vi "simulator.vi"() -> ()   [LabVIEW 2020]
doc: "This example demonstrates how to continuously acquire buffered voltage measurements using a DAQmx device.\n\nFor instructions on how to connect your signals to the DAQ device, refer to your device documentation."
uses:
  <vilib>/Utility/error.llb/DialogType.ctl
  <vilib>/measure/NI_MAPro.lvlib
  <vilib>/express/express arith-compare/Formula/XNode/ExpressFormulaBlockNode.xnode
  <vilib>/DAQmx/configure/task.llb/DAQmx Configure Logging (TDMS).vi
  <vilib>/measure/maspectr.llb/FFT Power Spectrum and PSD for N Chan.vi
  <vilib>/DAQmx/read.llb/DAQmx Read (Analog 1D Wfm NChan NSamp).vi
  <vilib>/express/express shared/transition.llb/Dynamic To Waveform Array.vi
  <vilib>/express/express arith-compare/Formula/Block/exnFormulaBlock how many pts in the wave.vi
  <vilib>/express/express shared/ex_Modify Signal Name.vi
  <vilib>/express/express shared/transition.llb/Waveform Array To Dynamic.vi
panel:
  in  "라디오 버튼":T1(radio)
  out "Sensor A Raw 6":dynamicdata(graph)
  in  "Sensor C Channel 2":tag="Dev2/ai0"
  in  "Sensor D Channel 2":tag="Dev2/ai1"
  in  "Terminal config 2":i32(ring)=10083 items=["default"=-1, "RSE"=10083, "NRSE"=10078, "Differential"=10106, "Pseudodifferential"=12529]
  out "A,B Filtering Signal 2":dynamicdata(graph)
  out "불리언 5":bool
  out "불리언 4":bool
  out "불리언 3":bool
  out "불리언 2":bool
  out "A,B Filtering Signal":dynamicdata(graph)
  out "Sensor A Raw 5":dynamicdata(graph)
  out "B Raw Signal":waveform(dbl)(graph)
  out "A Raw Signal":waveform(dbl)(graph)
  in  "TDMS File Path":path
  in  "Logging Mode":i32(ring)=10231 items=["Off"=10231, "Log and Read"=15842]
  in  "Sensor B Channel":tag="Dev2/ai1"
  in  "Sensor A Channel":tag="Dev2/ai0"
  in  "Terminal config":i32(ring)=10083 items=["default"=-1, "RSE"=10083, "NRSE"=10078, "Differential"=10106, "Pseudodifferential"=12529]
  in  "rate":dbl=5000.0
  out "FFT Power Spectrum":cluster{"f0":dbl, "df":dbl, "magnitude":dbl[]}[](graph)
  in  "Stop":bool
  in  "Number of Samples":i32=100
  # "A신호"
  # "B신호"
  # "Channel Settings"
  # "A신호"
  # "B신호"
  # "Logging Settings"
  # "A-B Signal Display"
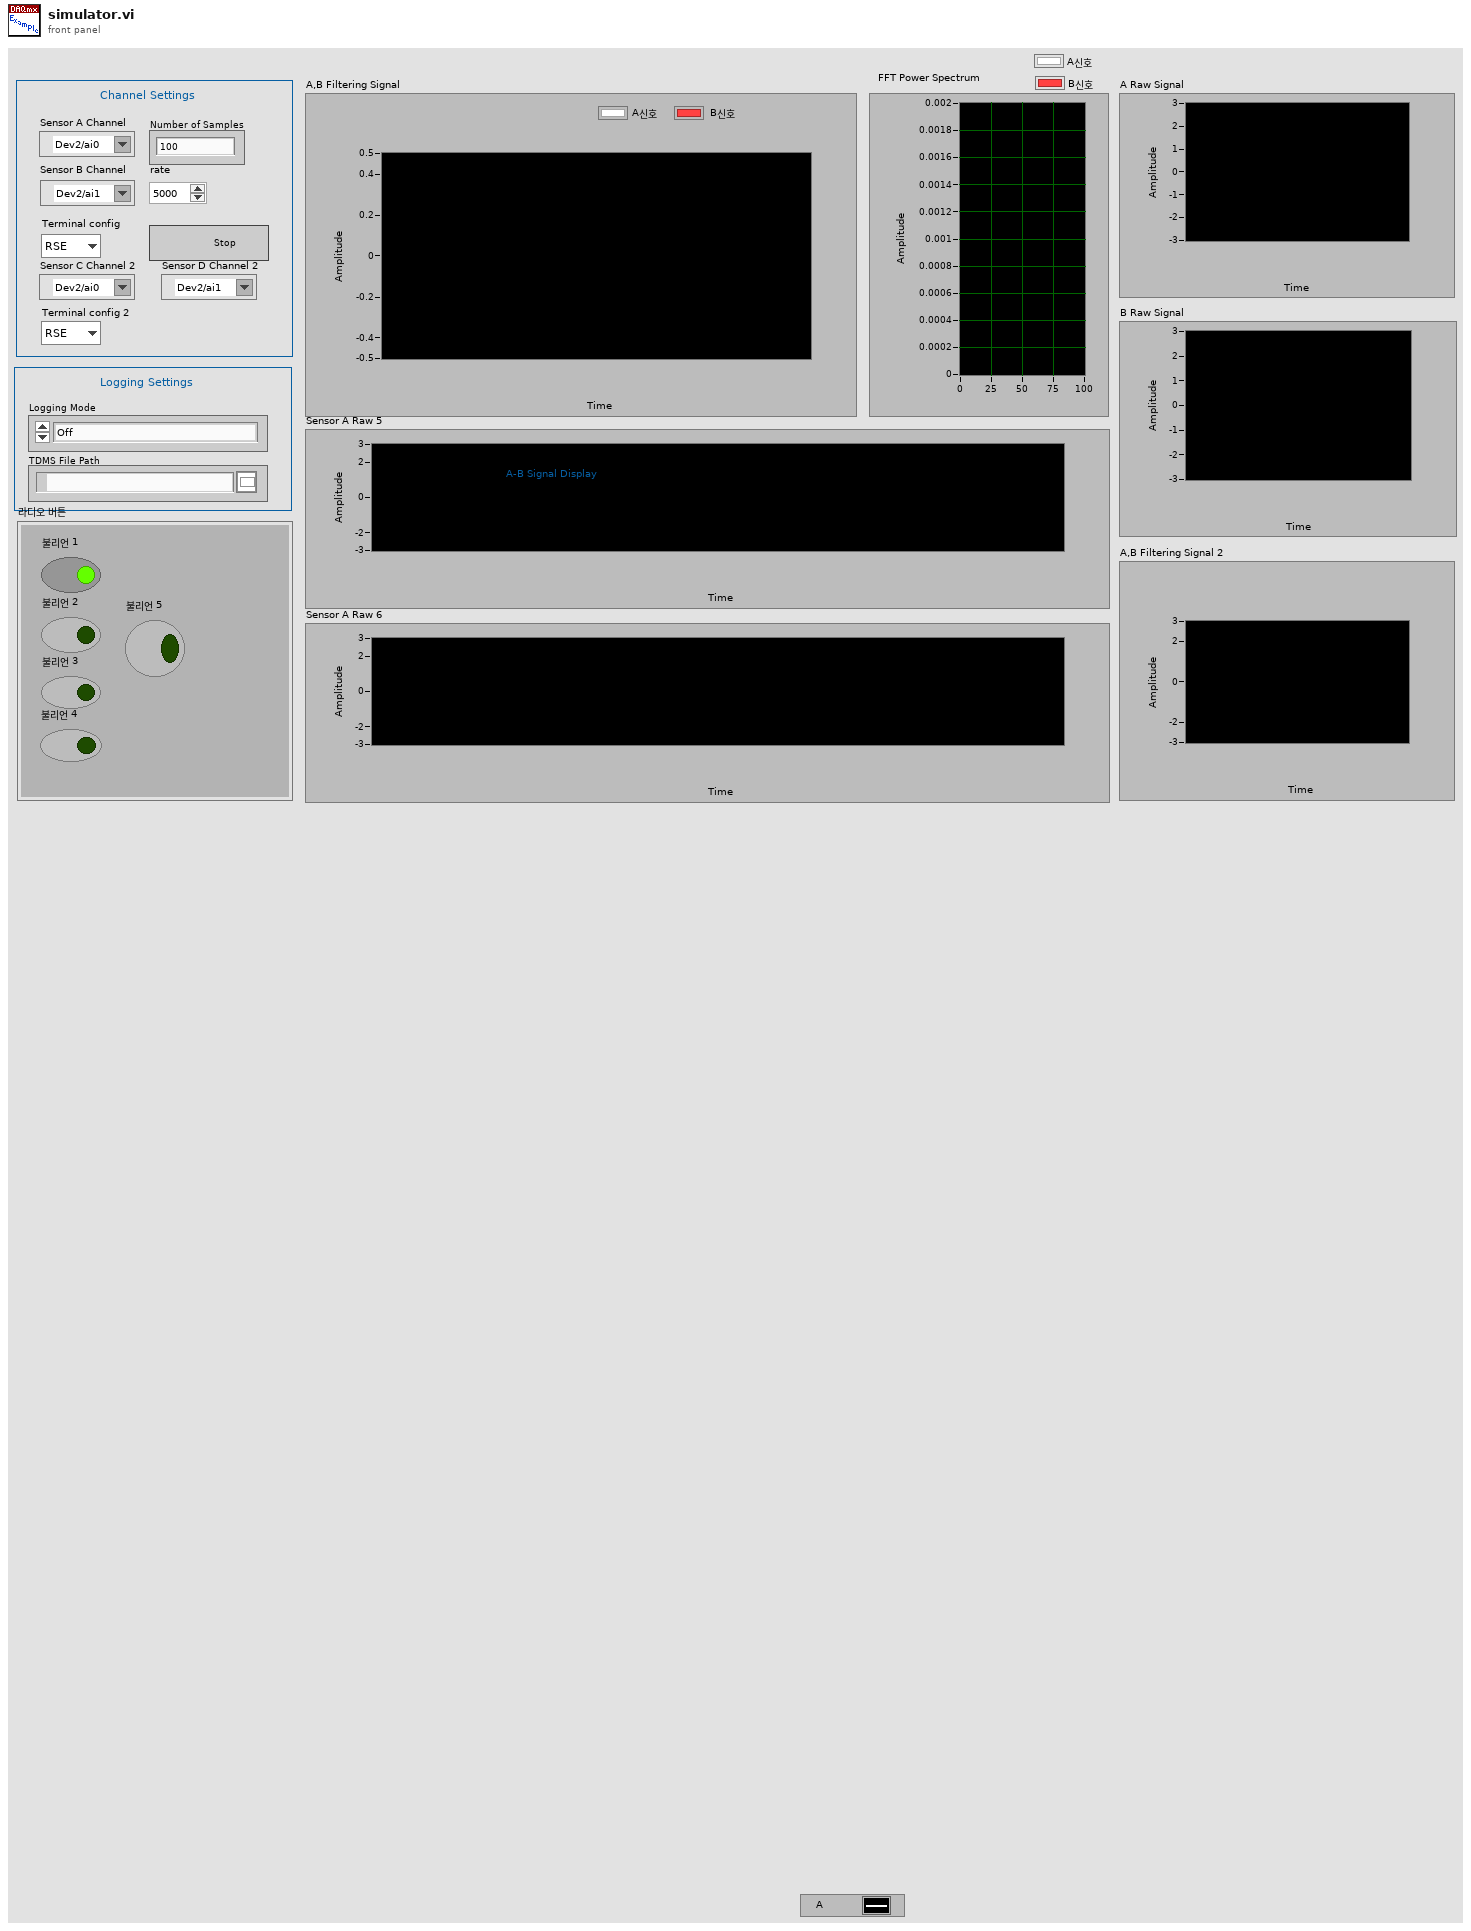
[diagram p1: front panel]
types:
  T1 = enum32{"불리언 1", "불리언 2", "불리언 3", "불리언 4", "불리언 5"}
  T2 = typedef "DialogType.ctl" = u16
  T3 = cluster{"averaging mode":enum16{"No averaging", "Vector averaging", "RMS averaging", "Peak hold"}, "weighting mode":enum16{"Linear", "Exponential"}, "number of averages":u32}
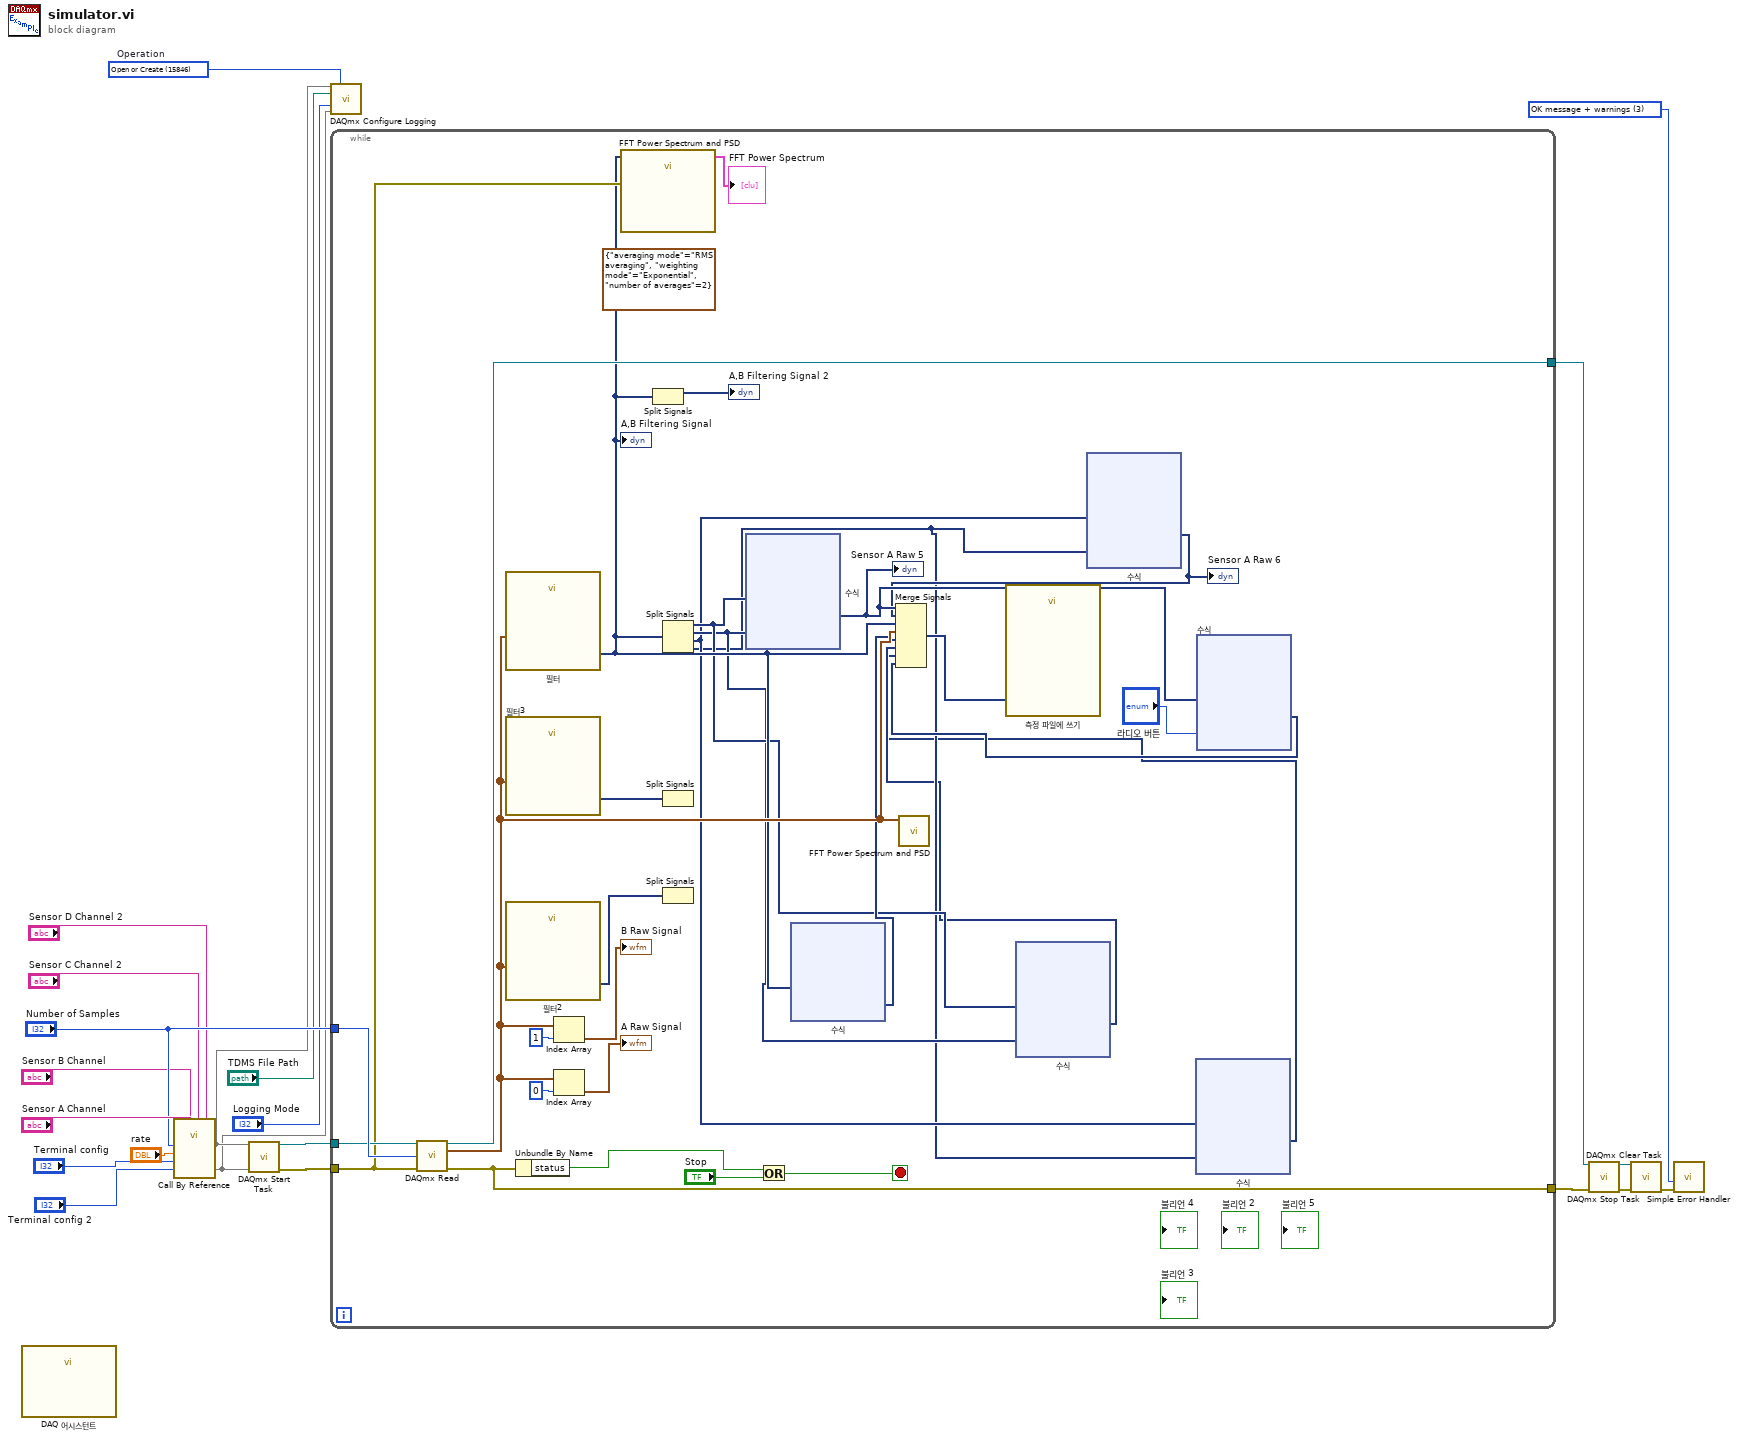
[diagram p0: block diagram]
diagram:
  w10 = 15846 items=["Open"=10437, "Open or Create"=15846, "Create or Replace"=15847, "Create"=15848]  # Operation
  w14 = T2 3 items=["no dialog", "OK message", "continue or stop message", "OK message + warnings", "continue/stop + warnings"] ("type of dialog (OK msg:1)")
  n1 = call "DAQ 어시스턴트"() -> ()  [unwired: 12 in]
  n2 = call-by-ref "?"(2:"Sensor D Channel 2", 5:"Sensor C Channel 2", 6:"Sensor A Channel", 7:"Sensor B Channel", 8:"Terminal config 2", 9:"Terminal config", 10:"rate", 11:"Number of Samples") -> (0:w6, 3:w7)  [unwired: 4 in, 2 out]
  n3 = call <vilib>:"DAQmx Start Task.vi"("task/channels in"=w7, "error in"=w6) -> ("task out"=w21:refnum<k21>, "error out"=w20:errorcluster)  [unwired: 12 in]
  n4 = call-poly <vilib>:"DAQmx Configure Logging.vi"("task/channels in"=w7, "operation"=w10, "file path"="TDMS File Path", "logging mode"="Logging Mode", "error in"=w6) -> ()  [unwired: 9 in, 2 out]
  n5 = while {
    tunnel: w21 -> [w45]
    tunnel: w20 -> [w44]
    tunnel: [w51] -> w18
    tunnel: [w49] -> w17
    tunnel: "Number of Samples" -> [w46]
    stop <- w47 stop-if-true
    (unwired) T3 {"averaging mode"=enum."RMS averaging", "weighting mode"=enum."Exponential", "number of averages"=2} ("averaging parameters")
    n6 = call-poly <vilib>:"DAQmx Read.vi"("task/channels in"=w45, "number of samples per channel"=w46, "error in"=w44) -> ("task out"=w51:refnum<k21>, "data"=w31:waveform(dbl)[], "error out"=w49:errorcluster)  [unwired: 10 in]
    n7 = call "필터"("Signal"=w31) -> ("Filtered Signal"=w29:dynamicdata)  [unwired: 9 in, 1 out]
    "A,B Filtering Signal" <- w29
    n8 = call "필터3"("Signal"=w31) -> ("Filtered Signal"=w36:dynamicdata)  [unwired: 9 in, 1 out]
    n9 = call "필터2"("Signal"=w31) -> ("Filtered Signal"=w37:dynamicdata)  [unwired: 9 in, 1 out]
    n10 = Unbundle By Name(w49) -> ("status"=w48:bool)
    n11 = Index Array(array=w31, index=1) -> (element=→"B Raw Signal":waveform(dbl))
    n12 = Index Array(array=w31, index=0) -> (element=→"A Raw Signal":waveform(dbl))
    n13 = call-poly <vilib>:"FFT Power Spectrum and PSD.vi"("error in (no error)"=w44, "time signals"=w29) -> ("Power Spectrum / PSD"=→"FFT Power Spectrum":cluster{"f0":dbl, "df":dbl, "magnitude":dbl[]}[])  [unwired: 6 in, 3 out]
    n14 = Split Signals(w29) -> (→"A,B Filtering Signal 2":dynamicdata)  [unwired: 2 in, 1 out]
    n15 = Split Signals(w29) -> (w27:dynamicdata, w26:dynamicdata, w25:dynamicdata, w24:dynamicdata)  [unwired: 4 in]
    n16 = Split Signals(w36) -> ()  [unwired: 2 in, 2 out]
    n17 = Split Signals(w37) -> ()  [unwired: 2 in, 2 out]
    n18 = xnode "수식"("X1"=w27, "X2"=w26) -> ("결과"=w33:dynamicdata)  [unwired: 1 in, 1 out]
    "Sensor A Raw 5" <- w33
    n19 = Or(x=w48, y="Stop") -> (x .or. y?=w47:bool)
    n20 = xnode "수식"("X1"=w29) -> ("결과"=w28:dynamicdata)  [unwired: 1 in, 1 out]
    n21 = call-poly <vilib>:"FFT Power Spectrum and PSD.vi"("time signals"=w31) -> ()  [unwired: 7 in, 4 out]
    n22 = xnode "수식"("X1"=w27, "X2"=w26) -> ("결과"=w23:dynamicdata)  [unwired: 1 in, 1 out]
    n23 = xnode "수식"("X1"=w25, "X2"=w24) -> ("결과"=w32:dynamicdata)  [unwired: 1 in, 1 out]
    "Sensor A Raw 6" <- w32
    n24 = xnode "수식"("X1"=w25, "X2"=w24) -> ("결과"=w22:dynamicdata)  [unwired: 1 in, 1 out]
    n25 = xnode "수식"("X1"=w33, "X2"="라디오 버튼") -> ("결과"=w30:dynamicdata)  [unwired: 1 in, 1 out]
    n26 = Merge Signals(w33, w32, w29, w31, w28, w23, w22, w30) -> (w38:dynamicdata)
    n27 = call "측정 파일에 쓰기"("Signals"=w38) -> ()  [unwired: 16 in, 3 out]
  }
  n28 = call <vilib>:"DAQmx Stop Task.vi"("task/channels in"=w18, "error in"=w17) -> ("task out"=w15:refnum<k21>, "error out"=w16:errorcluster)  [unwired: 12 in]
  n29 = call <vilib>:"DAQmx Clear Task.vi"("task in"=w15, "error in"=w16) -> ("error out"=w19:errorcluster)  [unwired: 13 in]
  n30 = call <vilib>:"Simple Error Handler.vi"("type of dialog (OK msg:1)"=w14, "error in (no error)"=w19) -> ()  [unwired: 3 in, 5 out]
